vi "getClaseVarilla.vi"(8 "error in":errorcluster, 11 "claseVarilla in":refnum<class "claseVarilla.lvclass">) -> (0 "error out":errorcluster, 2 "dataReading":T1, 3 "claseVarilla out":refnum<class "claseVarilla.lvclass">)   [LabVIEW 2014, in "claseVarilla.lvclass"]
uses:
  claseVarilla.lvclass
  claseVarilla.lvclass/claseVarilla.ctl
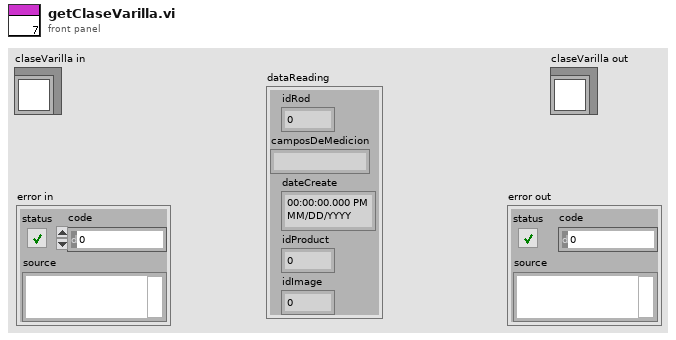
[diagram p1: front panel]
types:
  T1 = cluster{"idRod":dbl, "camposDeMedicion":string, "dateCreate":timestamp, "idProduct":dbl, "idImage":dbl}
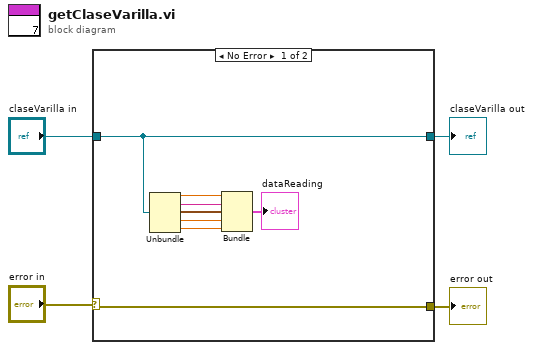
[diagram p0: block diagram]
diagram:
  n1 = case shown="No Error" "error in" {
    selector: "error in" -> [w12 w14]
    tunnel: [w12 w14] -> w3
    tunnel: "claseVarilla in" -> [w5 w13]
    tunnel: [w5 w13] -> w1
    frame No Error {
      n2 = Unbundle(w5) -> (w11:dbl, w10:string, w9:timestamp, w8:dbl, w7:dbl)
      n3 = Bundle("idRod"=w11, "camposDeMedicion"=w10, "dateCreate"=w9, "idProduct"=w8, "idImage"=w7) -> (→"dataReading":T1)  [unwired: 1 in]
    }
    frame Error {
    }
  }
  "claseVarilla out" <- w1
  "error out" <- w3
